vi "SaveReadImage2.vi"() -> ()   [LabVIEW 2014]
uses:
  <vilib>/picture/picture.llb/Draw True-Color Pixmap.vi
panel:
  out "new picture":picture
  out "new picture 2":picture
  out "error out":errorcluster
  in  "file path":path
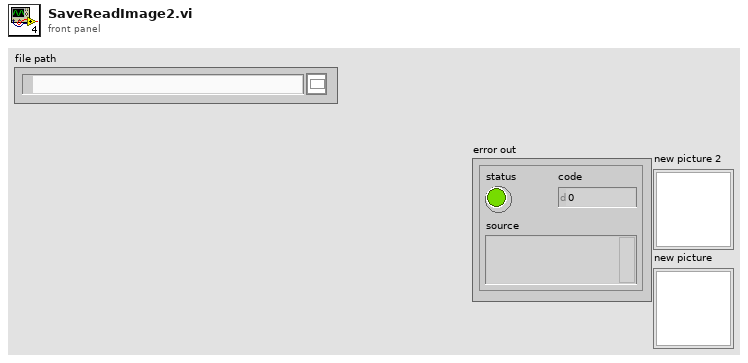
[diagram p1: front panel]
types:
  T1 = enum16{"open", "open or create", "create or replace", "create", "open (read-only)"}
  T2 = typedef "imagedata.ctl" = cluster{"image type":i32, "image depth":i32, "image":u8[], "mask":u8[], "colors":u32[], "Rectangle":cluster{"left":i16, "top":i16, "right":i16, "bottom":i16}}
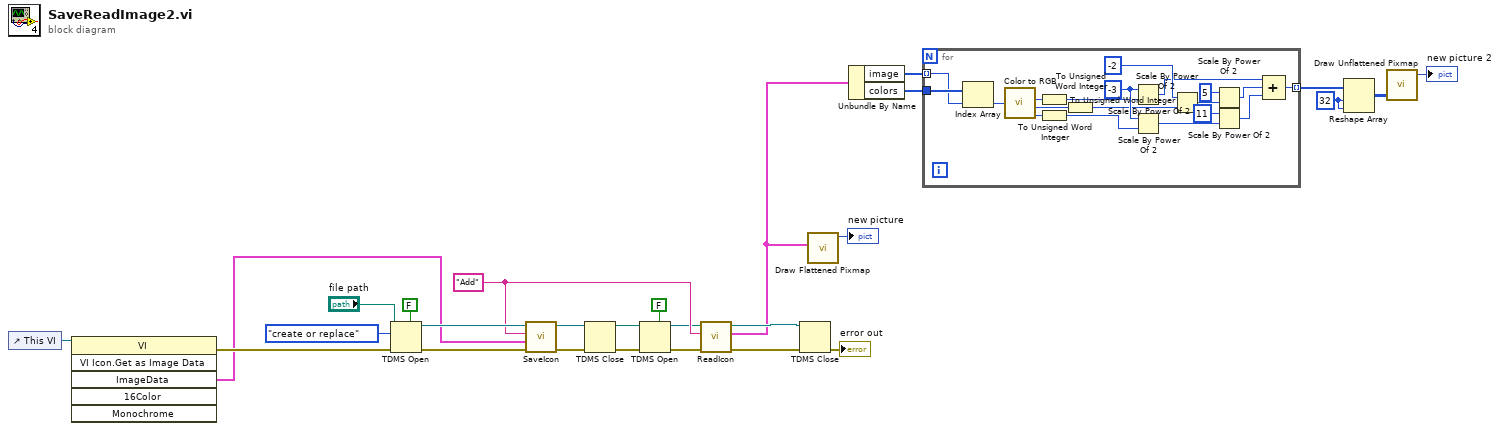
[diagram p0: block diagram]
diagram:
  w17 = 32 ("dimension size")
  w6 = "Add" ("group name in (Untitled)")
  n1 = control-ref of="This VI"() -> (w13:refnum<vi>)
  n2 = invoke class="VI" method="VI Icon.Get as Image Data"(reference=w13) -> (error out=w14:errorcluster, "ImageData"=w8:T2)  [unwired: 5 in, 4 out]
  n3 = TDMS Open(5:FALSE ("create index file? (T)"), 8:w14, 10:T1."create or replace" ("operation (0:open)"), 11:"file path") -> (0:w12:errorcluster, 3:w11:refnum<k34>)  [unwired: 3 in]
  n4 = call "SaveIcon.vi"("error in (no error)"=w12, "Icon"=w8, "Function"=w6, "TdmsIn"=w11) -> ("error out"=w10:errorcluster, "TdmsOuit"=w9:refnum<k34>)  [unwired: 6 in]
  n5 = TDMS Close(8:w10, 11:w9) -> (0:w7:errorcluster, 3:w27:path)
  n6 = TDMS Open(5:FALSE ("create index file? (T)"), 8:w7, 11:w27) -> (0:w5:errorcluster, 3:w4:refnum<k34>)  [unwired: 4 in]
  n7 = call "ReadIcon.vi"("error in (no error)"=w5, "Function"=w6, "TdmsIn"=w4) -> ("error out"=w3:errorcluster, "Icon"=w1:T2, "TdmsOut"=w2:refnum<k34>)  [unwired: 6 in]
  n8 = TDMS Close(8:w3, 11:w2) -> (0:→"error out":errorcluster)  [unwired: 1 out]
  n9 = call <vilib>:"Draw Flattened Pixmap.vi"("image data"=w1) -> ("new picture"=→"new picture":picture)  [unwired: 8 in]
  n10 = Unbundle By Name(w1) -> ("image"=w20:u8[], "colors"=w19:u32[])
  n11 = for {
    tunnel: w20 -> [w45] mode=indexing
    tunnel: w19 -> [w46]
    tunnel: [w30] -> w18 mode=indexing
    w43 = i16 -3 ("n")
    n12 = Index Array(array=w46, index=w45) -> (element=w44:u32)
    n13 = call <vilib>:"Color to RGB.vi"("Color"=w44) -> ("R"=w39:u8, "G"=w38:u8, "B"=w36:u8)  [unwired: 1 out]
    n14 = To Unsigned Word Integer(number=w39) -> (unsigned 16bit integer=w28:u16)
    n15 = To Unsigned Word Integer(number=w36) -> (unsigned 16bit integer=w29:u16)
    n16 = To Unsigned Word Integer(number=w38) -> (unsigned 16bit integer=w37:u16)
    n17 = Scale By Power Of 2(n=w43, x=w28) -> (x*2^n=w33:u16)
    n18 = Scale By Power Of 2(n=w43, x=w29) -> (x*2^n=w35:u16)
    n19 = Scale By Power Of 2(n=i16 -2, x=w37) -> (x*2^n=w41:u16)
    n20 = Scale By Power Of 2(n=i16 5, x=w41) -> (x*2^n=w32:u16)
    n21 = Scale By Power Of 2(n=i16 11, x=w35) -> (x*2^n=w31:u16)
    n22 = Compound Arithmetic op=ADD(w33, w32, w31) -> (w30:u16)
  }
  n23 = Reshape Array(w18, w17, w17) -> (w16:u16[][])
  n24 = call-poly <vilib>:"Draw Unflattened Pixmap.vi"("data (RGB format)"=w16) -> ("new picture"=→"new picture 2":picture)  [unwired: 8 in]
